vi "main_clear_environment.vi"(6 "Env. Clear":refnum<vi>, 9 "Env. ready?":refnum<vi>, 10 "Env. Dir":refnum<vi>, 11 "Env. Tree":refnum<vi>) -> ()   [LabVIEW 2019]
panel:
  # "*******************************************************************\nBiogas Plant Control\n\nAuthor: Paul Zügel\nGCSC-Frankfurt am Main 2020\n\n*******************************************************************"
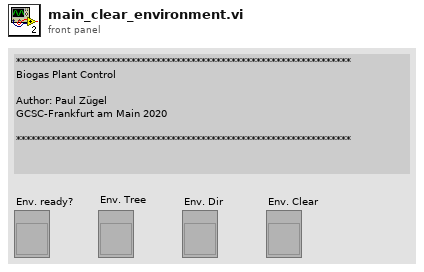
[diagram p1: front panel]
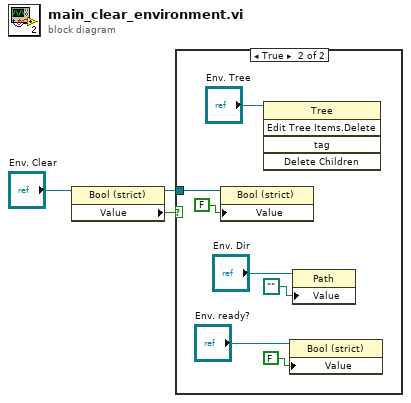
[diagram p0: block diagram]
diagram:
  n1 = property class="Bool (strict)"(reference="Env. Clear") -> (reference out=w1:refnum<vi>, "Value"=w2:bool)  [unwired: 1 in, 1 out]
  n2 = case shown="True" w2 {
    tunnel: w1 -> [_ w10]
    frame False {
    }
    frame True {
      n3 = property class="Bool (strict)"(reference=w10, "Value"=FALSE) -> ()  [unwired: 1 in, 2 out]
      n4 = invoke class="Tree" method="Edit Tree Items.Delete"(reference="Env. Tree") -> ()  [unwired: 4 in, 5 out]
      n5 = property class="Bool (strict)"(reference="Env. ready?", "Value"=FALSE) -> ()  [unwired: 1 in, 2 out]
      n6 = property class="Path"(reference="Env. Dir", "Value"=path "") -> ()  [unwired: 1 in, 2 out]
    }
  }
